vi "Set Data Test.vi"(8 "error in (no error)":errorcluster caption="entrée d'erreur (pas d'erreur)", 10 "Data_Test Read":T1(array[cluster]), 11 "Database Altyor en entrée":refnum<class "Database Altyor Packaging.lvclass">) -> (0 "error out":errorcluster caption="sortie d'erreur", 3 "Database Altyor en sortie":refnum<class "Database Altyor Packaging.lvclass">)   [LabVIEW 2020, in "Library Instrument & Equipement.lvlib" / "Library Database.lvlib" / "Database Altyor Packaging.lvclass"]
uses:
  Database Altyor Packaging.lvclass
  Database Altyor Packaging.lvclass/Database Altyor Packaging.ctl
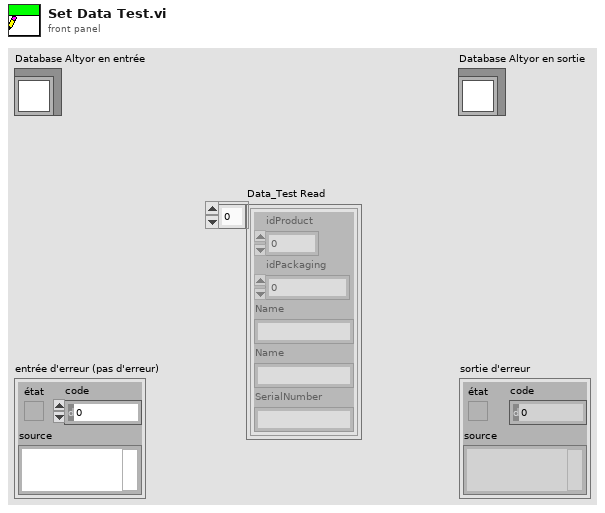
[diagram p1: front panel]
types:
  T1 = cluster{"idProduct":u32, "idPackaging":u32, "Name":string, "Name":string, "SerialNumber":string}[]
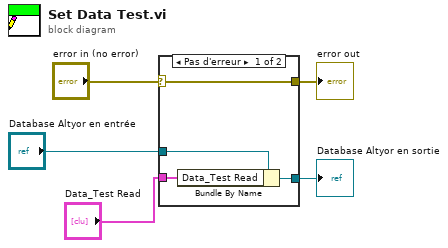
[diagram p0: block diagram]
diagram:
  n1 = case shown="Pas d'erreur" "error in (no error)" {
    selector: "error in (no error)" -> [w9 w10]
    tunnel: [w9 w10] -> w4
    tunnel: [w7 w11] -> w2
    tunnel: "Database Altyor en entrée" -> [w8 w11]
    tunnel: "Data_Test Read" -> [w6 _]
    frame No Error {
      n2 = Bundle By Name(cluster=w8, "Data_Test Read"=w6) -> (w7:refnum<class "Database Altyor Packaging.lvclass">)
    }
    frame Error {
    }
  }
  "error out" <- w4
  "Database Altyor en sortie" <- w2
